vi "missle move.vi"(10 "number of missles":i32, 11 "missles position in":cluster{i32, i32, i32}[](array[cluster])) -> (2 "new number of missles":i32, 3 "new missle position":cluster{i32, i32, i32}[](array[cluster]))   [LabVIEW 2019]
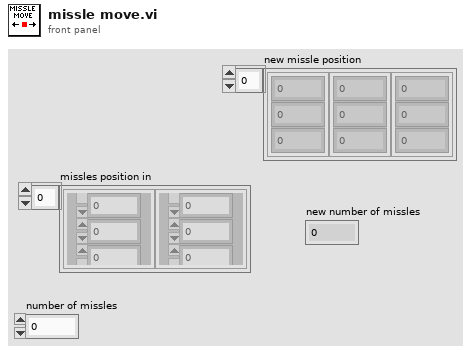
[diagram p1: front panel]
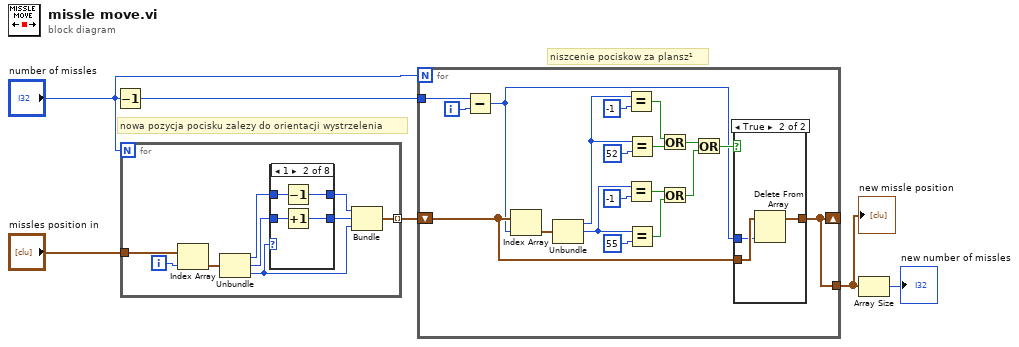
[diagram p0: block diagram]
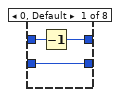
[diagram p3: hidden frame]
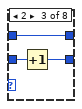
[diagram p4: hidden frame]
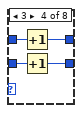
[diagram p5: hidden frame]
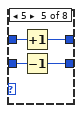
[diagram p6: hidden frame]
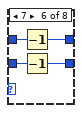
[diagram p7: hidden frame]
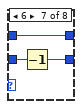
[diagram p8: hidden frame]
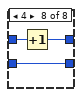
[diagram p9: hidden frame]
diagram:
  # "niszcenie pociskow za plansz¹"
  # "nowa pozycja pocisku zalezy do orientacji wystrzelenia"
  n1 = Decrement(x="number of missles") -> (x-1=w5:i32)
  n2 = for {
    N: "number of missles" -> [_]
    tunnel: "missles position in" -> [w9]
    tunnel: [w10] -> w3 mode=indexing
    i -> [w8]
    n3 = Index Array(array=w9, index=w8) -> (element=w7:cluster{i32, i32, i32})
    n4 = Unbundle(w7) -> (w15:i32, w14:i32, w13:i32)
    n5 = case shown="1" w13 {
      tunnel: w14 -> [w18 w22 w25 w29 w33 w37 w40 w42]
      tunnel: w15 -> [w17 w21 w24 w28 w32 w36 w39 w43]
      tunnel: [w18 w20 w23 w27 w30 w35 w38 w42] -> w12
      tunnel: [w16 w19 w24 w26 w31 w34 w39 w41] -> w11
      frame 0, Default {
        n6 = Decrement(x=w17) -> (x-1=w16:i32)
      }
      frame 1 {
        n7 = Decrement(x=w21) -> (x-1=w19:i32)
        n8 = Increment(x=w22) -> (x+1=w20:i32)
      }
      frame 2 {
        n9 = Increment(x=w25) -> (x+1=w23:i32)
      }
      frame 3 {
        n10 = Increment(x=w28) -> (x+1=w26:i32)
        n11 = Increment(x=w29) -> (x+1=w27:i32)
      }
      frame 5 {
        n12 = Increment(x=w32) -> (x+1=w31:i32)
        n13 = Decrement(x=w33) -> (x-1=w30:i32)
      }
      frame 7 {
        n14 = Decrement(x=w36) -> (x-1=w34:i32)
        n15 = Decrement(x=w37) -> (x-1=w35:i32)
      }
      frame 6 {
        n16 = Decrement(x=w40) -> (x-1=w38:i32)
      }
      frame 4 {
        n17 = Increment(x=w43) -> (x+1=w41:i32)
      }
    }
    n18 = Bundle(w11, w12, w13) -> (w10:cluster{i32, i32, i32})  [unwired: 1 in]
  }
  n19 = for {
    N: "number of missles" -> [_]
    shift-right: [w45] -> _
    shift-left: w3 -> [w48]
    tunnel: [w45] -> w2
    tunnel: w5 -> [w44]
    i -> [w49]
    n20 = Subtract(x=w44, y=w49) -> (x-y=w46:i32)
    n21 = Index Array(array=w48, index=w46) -> (element=w47:cluster{i32, i32, i32})
    n22 = Unbundle(w47) -> (w61:i32, w56:i32)  [unwired: 1 out]
    n23 = Equal?(x=w61, y=-1) -> (x = y?=w59:bool)
    n24 = Equal?(x=w56, y=-1) -> (x = y?=w54:bool)
    n25 = Equal?(x=w61, y=52) -> (x = y?=w58:bool)
    n26 = Equal?(x=w56, y=55) -> (x = y?=w53:bool)
    n27 = Or(x=w59, y=w58) -> (x .or. y?=w52:bool)
    n28 = Or(x=w54, y=w53) -> (x .or. y?=w51:bool)
    n29 = Or(x=w52, y=w51) -> (x .or. y?=w50:bool)
    n30 = case shown="True" w50 {
      tunnel: w48 -> [w63 w66]
      tunnel: w46 -> [_ w65]
      tunnel: [w63 w64] -> w45
      frame False {
      }
      frame True {
        n31 = Delete From Array(array=w66, index=w65) -> (array with subset deleted=w64:cluster{i32, i32, i32}[])  [unwired: 1 in, 1 out]
      }
    }
  }
  "new missle position" <- w2
  n32 = Array Size(array=w2) -> (size(s)=→"new number of missles":i32)
